vi "Write Data Word Format.vi"(8 "error in (no error)":errorcluster, 10 "Data Word Format":T1, 11 "CSV Word Logger in":refnum<class "CSV Word Logger.lvclass">) -> (0 "error out":errorcluster, 3 "CSV Word Logger out":refnum<class "CSV Word Logger.lvclass">)   [LabVIEW 2020, in "AIM MIL-STD-1553 Engine.lvlib" / "Implementation.lvlib" / "CSV Word Logger.lvclass"]
uses:
  CSV Word Logger.lvclass
  Shared/Data Word Format.ctl
  CSV Word Logger.lvclass/CSV Word Logger.ctl
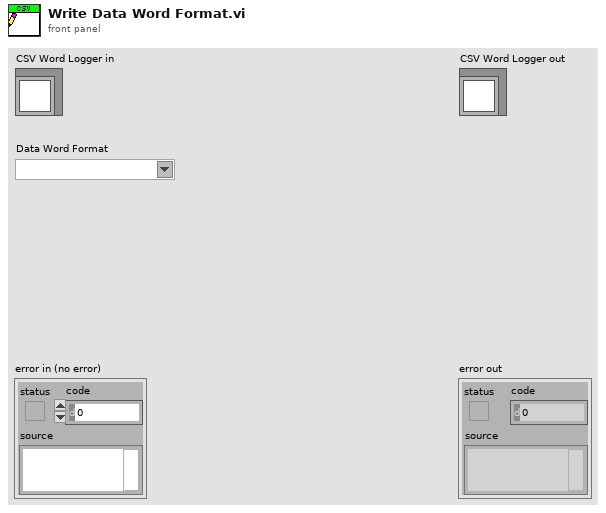
[diagram p1: front panel]
types:
  T1 = typedef "Data Word Format.ctl" = string
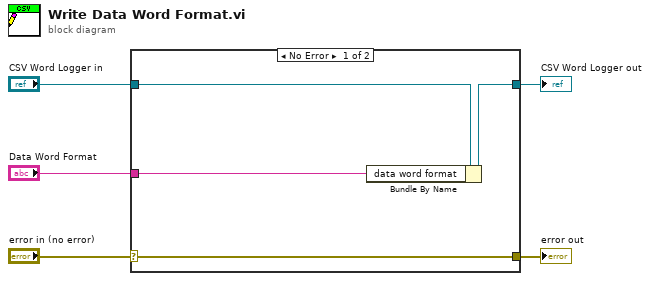
[diagram p0: block diagram]
diagram:
  n1 = case shown="No Error" "error in (no error)" {
    selector: "error in (no error)" -> [w9 w10]
    tunnel: [w9 w10] -> w4
    tunnel: [w6 w11] -> w2
    tunnel: "CSV Word Logger in" -> [w8 w11]
    tunnel: "Data Word Format" -> [w7 _]
    frame No Error {
      n2 = Bundle By Name(cluster=w8, "data word format"=w7) -> (w6:refnum<class "CSV Word Logger.lvclass">)
    }
    frame Error {
    }
  }
  "error out" <- w4
  "CSV Word Logger out" <- w2
